vi "Class to gRPC_to_Main.vi"(11 "Timed Node in":refnum<class "BTSTemplateTest.lvclass">) -> (2 "gRPC to Main":T1, 3 "Timed Node out":refnum<class "BTSTemplateTest.lvclass">)   [LabVIEW 2023, in "BTSTemplateTest.lvlib" / "BTSTemplateTest.lvclass"]
uses:
  BTSTemplateTest.lvclass
  Type Defs/gRPC to Main.ctl
  BTSTemplateTest.lvclass/BTSTemplateTest.ctl
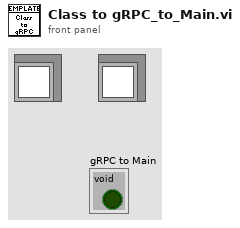
[diagram p1: front panel]
types:
  T1 = typedef "BTSTemplateTest.lvlib/BTSTemplateTest.lvclass/gRPC to Main.ctl" = cluster{"void":bool}
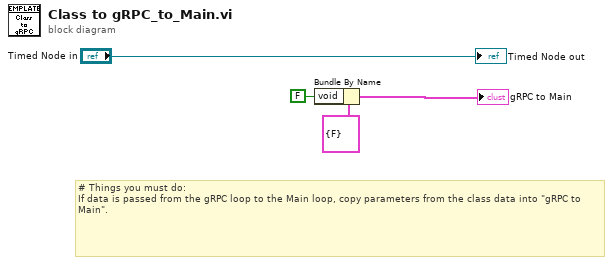
[diagram p0: block diagram]
diagram:
  # "# Things you must do:\nIf data is passed from the gRPC loop to the Main loop, copy parameters from the class data into \"gRPC to Main\"."
  n1 = Bundle By Name(cluster=T1 {"void"=FALSE} ("gRPC to Main"), "void"=FALSE) -> (→"gRPC to Main":T1)
  "Timed Node out" <- "Timed Node in"
